vi "Get Input List.vi"(8 "error in (no error)":errorcluster, 11 "OBS in":refnum<class "OBS.lvclass">) -> (0 "error out":errorcluster, 2 "Inputs":T1[](array[typedef]), 3 "OBS out":refnum<class "OBS.lvclass">)   [LabVIEW 2020, in "obs-websocket.lvlib" / "OBS.lvclass"]
uses:
  OBS.lvclass
  OBS.lvclass/OBS.ctl
  GetInputList/GetInputList.lvclass
  RGetInputList/RGetInputList.lvclass
  C:/dev/lv20CE/lv-obs-websocket/obs-websocket-lv/Response/Response.lvclass
  C:/dev/lv20CE/lv-obs-websocket/obs-websocket-lv/Server Message/Server Message.lvclass
  C:/dev/lv20CE/lv-obs-websocket/obs-websocket-lv/Message/Message.lvclass
  C:/dev/lv20CE/lv-obs-websocket/obs-websocket-lv/RGetInputList/RGetInputList.lvclass
  C:/dev/lv20CE/lv-obs-websocket/obs-websocket-lv/Request/Request.lvclass
  C:/dev/lv20CE/lv-obs-websocket/obs-websocket-lv/Client Message/Client Message.lvclass
  C:/dev/lv20CE/lv-obs-websocket/obs-websocket-lv/GetInputList/GetInputList.lvclass
  Input Settings.ctl
  obs-websocket.lvlib
  Input.ctl
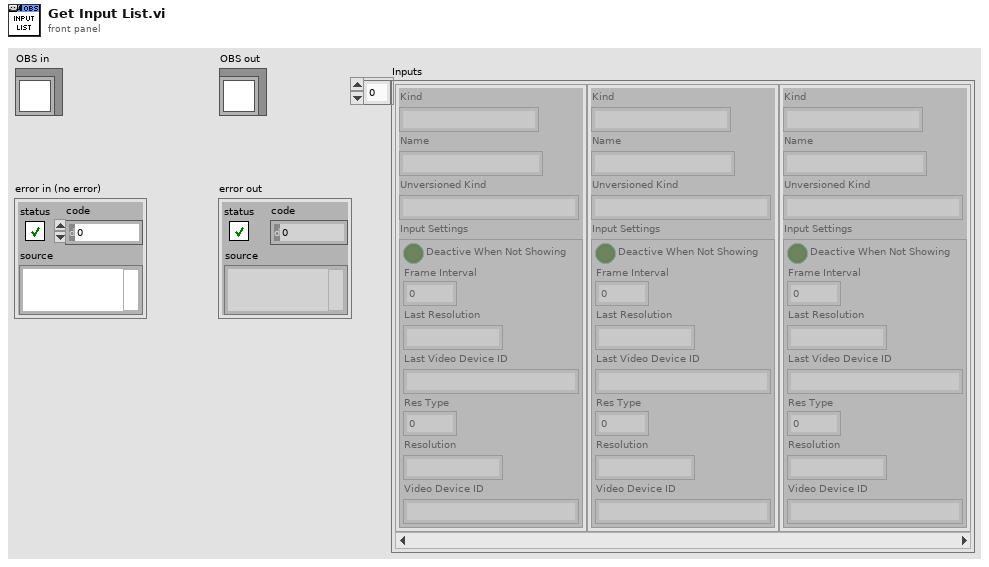
[diagram p1: front panel]
types:
  T1 = typedef "obs-websocket.lvlib/Input.ctl" = cluster{"Kind":string, "Name":string, "Unversioned Kind":string, "Input Settings":T2}
  T2 = typedef "obs-websocket.lvlib/Input Settings.ctl" = cluster{"Deactive When Not Showing":bool, "Frame Interval":i32, "Last Resolution":string, "Last Video Device ID":string, "Res Type":i32, "Resolution":string, "Video Device ID":string}
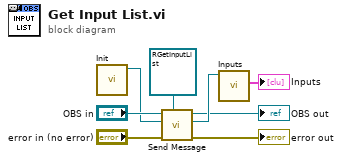
[diagram p0: block diagram]
diagram:
  n1 = call "Init.vi"() -> ("GetInputList out"=w6:refnum<class "GetInputList.lvclass">)  [unwired: 10 in, 1 out]
  n2 = call "Send Message.vi"("Response Type (None)"=refnum<class "RGetInputList.lvclass"> refnum ("obs-websocket-lv.lvlib:RGetInputList.lvclass"), "error in (no error)"="error in (no error)", "Client Message"=w6, "OBS in"="OBS in") -> ("error out"=→"error out":errorcluster, "Response Type (None)"=w4:refnum<class "RGetInputList.lvclass">, "OBS in"=→"OBS out":refnum<class "OBS.lvclass">)  [unwired: 4 in, 1 out]
  n3 = call "Inputs.vi"("RGetInputList in"=w4) -> ("Inputs"=→"Inputs":T1[])  [unwired: 8 in, 2 out]
